vi "TopLevel_menu tester.vi"() -> ()   [LabVIEW 2009]
panel:
  in  "Left buttons":T1
  in  "Options buttons":T2
  out "Menu item clicked?":bool
  in  "Stop Button":bool
  # "Click  the Left Menu or the Top Menu"
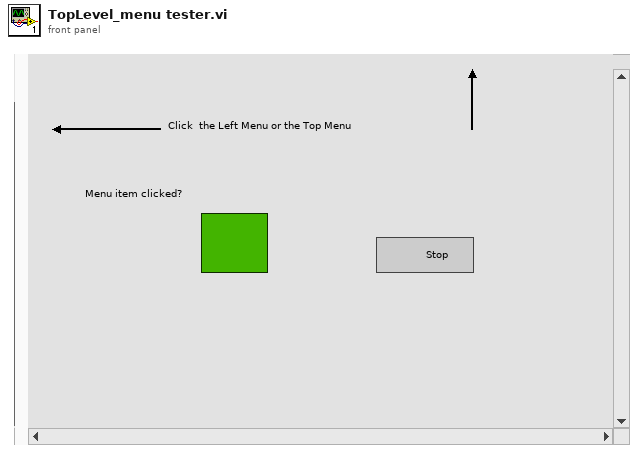
[diagram p1: front panel]
types:
  T1 = cluster{"New Button":bool, "Open Button":bool, "Save Button":bool, "Help Button":bool, "Search Button":bool}
  T2 = cluster{"Preferences Button":bool, "Settings Button":bool, "Lock Button":bool, "Add Button":bool}
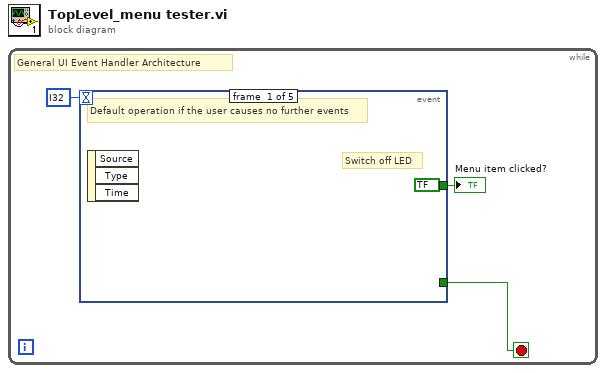
[diagram p0: block diagram]
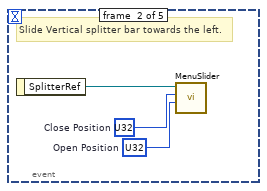
[diagram p2: hidden frame]
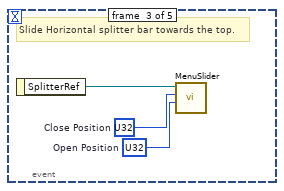
[diagram p3: hidden frame]
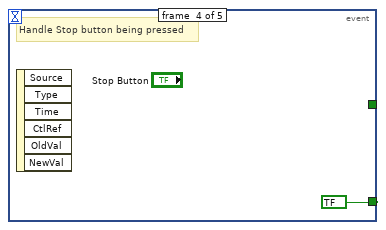
[diagram p4: hidden frame]
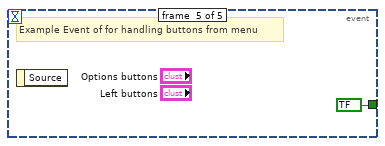
[diagram p5: hidden frame]
diagram:
  n1 = while {
    stop <- w3 stop-if-true
    # "General UI Event Handler Architecture"
    n2 = event shown="[1] \"Left menu\": Mouse Up" {
      selector: _ -> [_ _ _ _ _]
      dyn-events: _ -> [_ _ _ _ _]
      timeout: i32 ? -> [_ _ _ _ _]
      tunnel: [_ _ _ bool ? ("Stop Button") _] -> w3
      tunnel: [bool ? ("Stop Button") _ _ _ bool ? ("Stop Button")] -> w2
      event #0 {
        # "Switch off LED"
        # "Default operation if the user causes no further events"
        n3 = event-data() -> ()  [unwired: 1 in, 3 out]
      }
      event #1 {
        w5 = u32 ?  # Open Position
        w6 = u32 ?  # Close Position
        # "Slide Vertical splitter bar towards the left."
        n4 = event-data() -> ("SplitterRef"=w7:refnum<vi>)  [unwired: 1 in]
        n5 = call "MenuSlider.vi"("Open Position"=w5, "Close Position"=w6, "Splitter Refnum"=w7) -> ()  [unwired: 8 in, 1 out]
      }
      event #2 {
        w8 = u32 ?  # Open Position
        w9 = u32 ?  # Close Position
        # "Slide Horizontal splitter bar towards the top."
        n6 = event-data() -> ("SplitterRef"=w10:refnum<vi>)  [unwired: 1 in]
        n7 = call "MenuSlider.vi"("Open Position"=w8, "Close Position"=w9, "Splitter Refnum"=w10) -> ()  [unwired: 8 in, 1 out]
      }
      event #3 {
        # "Handle Stop button being pressed"
        n8 = event-data() -> ()  [unwired: 1 in, 6 out]
      }
      event #4 {
        # "Example Event of for handling buttons from menu"
        n9 = event-data() -> ()  [unwired: 1 in, 1 out]
      }
    }
    "Menu item clicked?" <- w2
  }
